vi "STOP.vi"(8 "error in (no error)":errorcluster, 11 "Stop in":refnum<class "DAQmxTaksContainer_Emulate.lvclass">) -> (0 "error out":errorcluster, 3 "Stop out":refnum<class "DAQmxTaksContainer_Emulate.lvclass">)   [LabVIEW 2015, in "DAQmxTaksContainer_Emulate.lvclass"]
uses:
  DAQmxTaksContainer_Emulate.lvclass
  DAQmxTaskContainer_General/DAQmxTaksContainer_General.lvclass
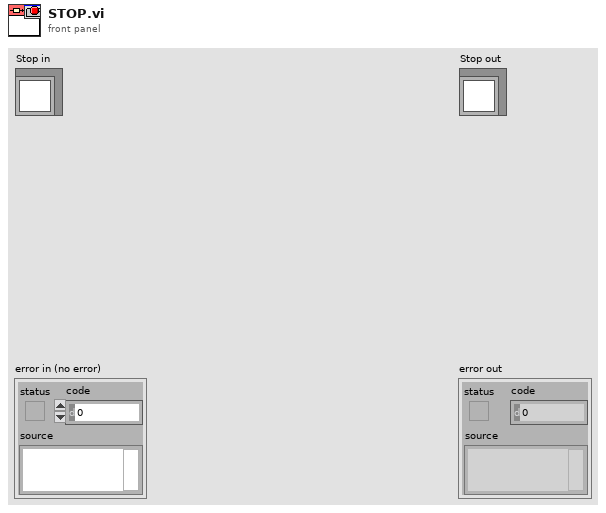
[diagram p1: front panel]
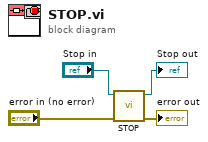
[diagram p0: block diagram]
diagram:
  n1 = call-parent "STOP.vi"("error in (no error)"="error in (no error)", "Stop in"="Stop in") -> ("error out"=→"error out":errorcluster, "Stop out"=→"Stop out":refnum<class "DAQmxTaksContainer_Emulate.lvclass">)  [unwired: 8 in]
